vi "自动删除过期数据文件.vi"(9 "保留文件个数":i32, 10 "最大文件个数":i32, 11 "文件夹路径":path) -> (2 "删除结果":T1)   [LabVIEW 2018]
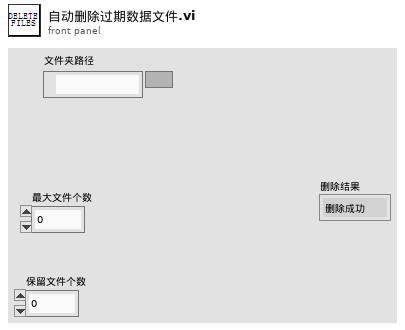
[diagram p1: front panel]
types:
  T1 = typedef "删除状态.ctl" = enum16{"删除成功", "删除出错"}
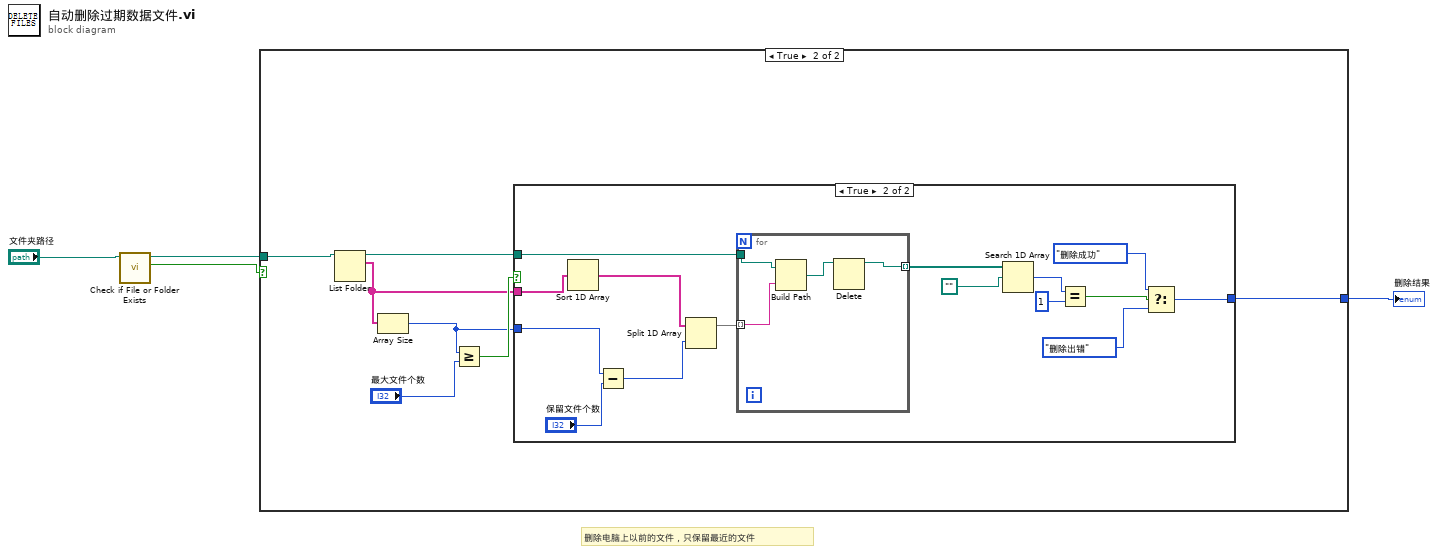
[diagram p0: block diagram]
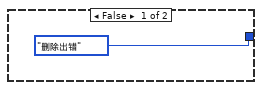
[diagram p2: hidden frame]
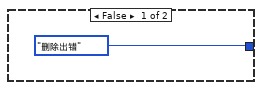
[diagram p3: hidden frame]
diagram:
  # "删除电脑上以前的文件，只保留最近的文件"
  n1 = call <vilib>:"Check if File or Folder Exists.vi"("path"="文件夹路径") -> ("file or folder exists?"=w3:bool, "dup path"=w2:path)  [unwired: 8 in, 1 out]
  n2 = case shown="True" w3 {
    tunnel: w2 -> [_ w12]
    tunnel: [删除状态."删除出错" ("f") w6] -> w1
    frame False {
    }
    frame True {
      n3 = List Folder(path=w12) -> (path out=w7:path, filenames=w9:string[])  [unwired: 3 in, 2 out]
      n4 = Array Size(array=w9) -> (size(s)=w8:i32)
      n5 = Greater Or Equal?(x=w8, y="最大文件个数") -> (x >= y?=w10:bool)
      n6 = case shown="True" w10 {
        tunnel: w9 -> [_ w28]
        tunnel: w8 -> [_ w26]
        tunnel: w7 -> [_ w22]
        tunnel: [删除状态."删除出错" ("f") w14] -> w6
        frame False {
        }
        frame True {
          n7 = Sort 1D Array(array=w28) -> (sorted array=w24:string[])
          n8 = Subtract(x=w26, y="保留文件个数") -> (x-y=w25:i32)
          n9 = Split 1D Array(array=w24, index=w25) -> (first subarray=w23:string[])  [unwired: 1 out]
          n10 = for {
            tunnel: w23 -> [w31] mode=indexing
            tunnel: w22 -> [w32]
            tunnel: [w29] -> w21 mode=indexing
            n11 = Build Path(base path=w32, name or relative path=w31) -> (appended path=w30:path)
            n12 = Delete(path (use dialog)=w30) -> (deleted path=w29:path)  [unwired: 4 in, 2 out]
          }
          n13 = Search 1D Array(1D array=w21, element=path "") -> (index of element=w19:i32)  [unwired: 1 in]
          n14 = Equal?(x=w19, y=1) -> (x = y?=w17:bool)
          n15 = Select(t=删除状态."删除成功" ("删除结果"), s=w17, f=删除状态."删除出错") -> (s? t:f=w14:T1)
        }
      }
    }
  }
  "删除结果" <- w1
